vi "LJM startup config.vi"(0 "Working Directory":path, 5 "App Name":string="ljstreamud.cfg") -> (1 "Data File Prefix":string="data", 2 "Scan Rate (Hz)":dbl=500.0 format="%.3f", 3 "Graph History":i32=1000 min=0, 4 "# Channels":i32=4, 6 "Disable Scaling":bool, 8 "Max File Size (Bytes)":i32=1048576, 9 "Write To File":bool, 10 "Channel Setup":T1={"+Ch"=["0", "1", "2", "3", "4", "5", "6", "7"], "-Ch"=["199", "199", "199", "199", "199", "199", "199", "199"], "Ranges"=[0, 0, 0, 0, 0, 0, 0, 0], "Scaling Equation"=["y=v0", "y=v1", "y=v2", "y=v3", "y=v4", "y=v5", "y=v6", "y=v7"], "Graph?"=[]} {"Ranges" items=["LJ_rgBIP10V", "LJ_rgBIP5V", "LJ_rgUNI5V", "LJ_rgUNI2P5V", "LJ_rgUNI1P25V", "LJ_rgBIP1V", "LJ_rgUNIP625V", "LJ_rgBIPP1V", "LJ_rgBIPP01V"]}, 12 "Interval (ms)":u32=500, 13 "Resolution":u8, 14 "SettlingFactor":u8, 15 "error out":errorcluster)   [LabVIEW 2025]
uses:
  LJstreamM globals.vi
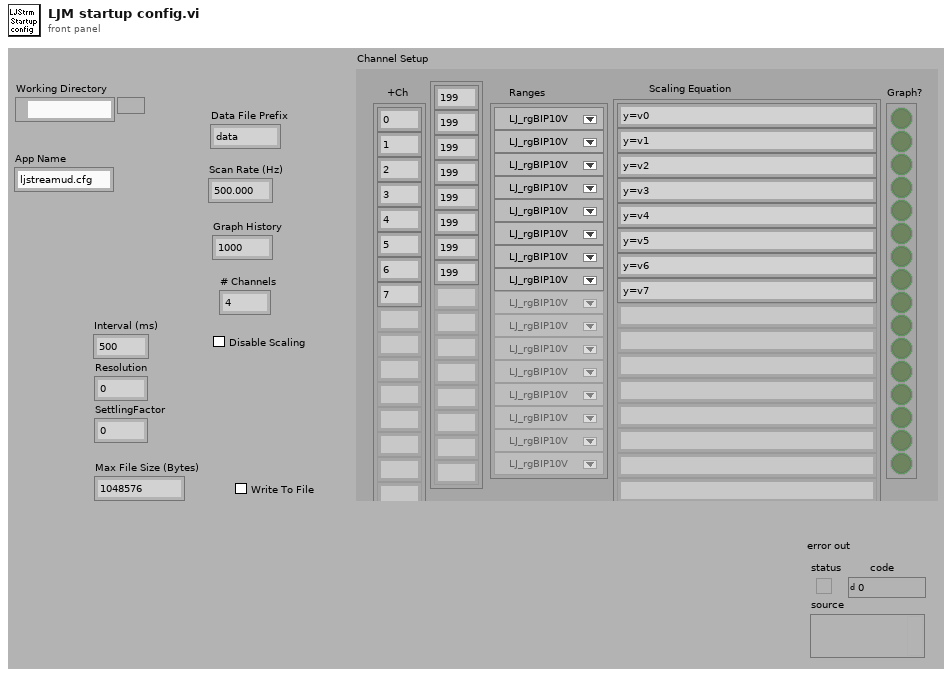
[diagram p1: front panel]
types:
  T1 = cluster{"+Ch":string[], "-Ch":string[], "Ranges":u16[], "Scaling Equation":string[], "Graph?":bool[]}
  T2 = cluster{"Data File Prefix":string, "Scan Rate (Hz)":dbl, "Graph History":i32, "# Channels":i32, "Disable Scaling":bool, "Max File Size (Bytes)":i32, "Channel Setup":cluster{"+Ch":string[], "-Ch":string[], "Ranges":u16[], "Scaling Equation":string[], "Graph?":bool[]}, "Interval (ms)":u32, "Write To File":bool}
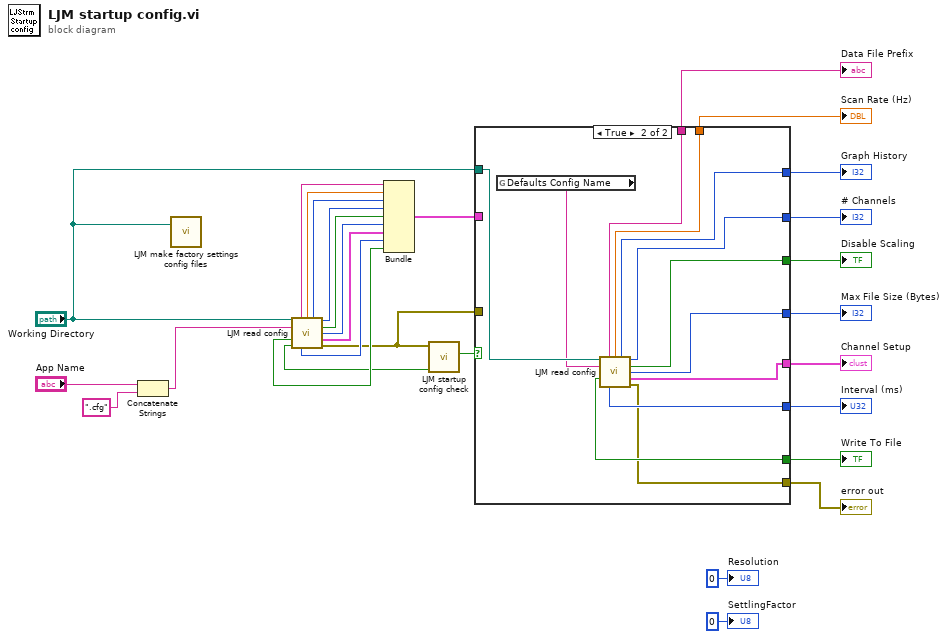
[diagram p0: block diagram]
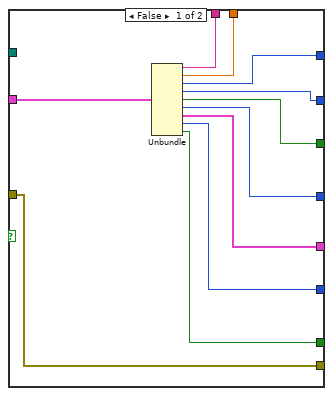
[diagram p2: hidden frame]
diagram:
  n1 = Concatenate Strings("App Name", ".cfg" ("string")) -> (w27:string)
  n2 = call "LJM make factory settings config files.vi"("Working Directory"="Working Directory") -> ()  [unwired: 3 in]
  n3 = call "LJM read config.vi"("Working Directory"="Working Directory", "filename"=w27) -> ("Data File Prefix"=w26:string, "Scan Rate (Hz)"=w25:dbl, "Graph History"=w24:i32, "# Channels"=w23:i32, "Disable Scaling"=w22:bool, "Max File Size (Bytes)"=w21:i32, "Write To File"=w18:bool, "Channel Setup"=w20:T1, "Good Experiment Config"=w17:bool, "Interval (ms)"=w19:u32, "error out"=w4:errorcluster)  [unwired: 1 in, 2 out]
  n4 = Bundle("Data File Prefix"=w26, "Scan Rate (Hz)"=w25, "Graph History"=w24, "# Channels"=w23, "Disable Scaling"=w22, "Max File Size (Bytes)"=w21, "Channel Setup"=w20, "Interval (ms)"=w19, "Write To File"=w18) -> (w15:T2)  [unwired: 1 in]
  n5 = call "LJM startup config check.vi"("Good Config?"=w17, "Config Error In"=w4) -> ("Force Defaults"=w16:bool)  [unwired: 9 in]
  n6 = case shown="True" w16 {
    tunnel: w15 -> [w40 _]
    tunnel: "Working Directory" -> [_ w52]
    tunnel: [w39 w50] -> w13
    tunnel: [w38 w49] -> w12
    tunnel: [w37 w48] -> w11
    tunnel: [w36 w47] -> w10
    tunnel: [w35 w46] -> w9
    tunnel: [w31 w45] -> w8
    tunnel: [w32 w44] -> w7
    tunnel: [w33 w43] -> w6
    tunnel: [w34 w42] -> w5
    tunnel: w4 -> [w30 _]
    tunnel: [w30 w41] -> w3
    frame False {
      n7 = Unbundle(w40) -> ("Data File Prefix"=w39:string, "Scan Rate (Hz)"=w38:dbl, "Graph History"=w37:i32, "# Channels"=w36:i32, "Disable Scaling"=w35:bool, "Max File Size (Bytes)"=w31:i32, "Channel Setup"=w32:T1, "Interval (ms)"=w33:u32, "Write To File"=w34:bool)
    }
    frame True {
      n8 = global read "LJstreamM globals.vi" "Defaults Config Name"() -> (w51:string)
      n9 = call "LJM read config.vi"("Working Directory"=w52, "filename"=w51) -> ("Data File Prefix"=w50:string, "Scan Rate (Hz)"=w49:dbl, "Graph History"=w48:i32, "# Channels"=w47:i32, "Disable Scaling"=w46:bool, "Max File Size (Bytes)"=w45:i32, "Write To File"=w42:bool, "Channel Setup"=w44:T1, "Interval (ms)"=w43:u32, "error out"=w41:errorcluster)  [unwired: 1 in, 3 out]
    }
  }
  "error out" <- w3
  "Channel Setup" <- w7
  "Interval (ms)" <- w6
  "Graph History" <- w11
  "# Channels" <- w10
  "Disable Scaling" <- w9
  "Data File Prefix" <- w13
  "Scan Rate (Hz)" <- w12
  "Max File Size (Bytes)" <- w8
  "Write To File" <- w5
  "SettlingFactor" <- u8 0 ("SettlingFactor")
  "Resolution" <- u8 0 ("Resolution")
